vi "comm termination.vi"(8 "error in (no error)":errorcluster, 9 "termination characters":string, 10 "Termination Character Enable":bool, 11 "Comm Handle":u32) -> (0 "error out":errorcluster, 3 "dup Comm Handle":u32)   [LabVIEW 2017, in "lvserial.lvlib"]
doc: "Configures the termiation characters for the serial port."
uses:
  lvserial.lvlib
  lvserial.dll
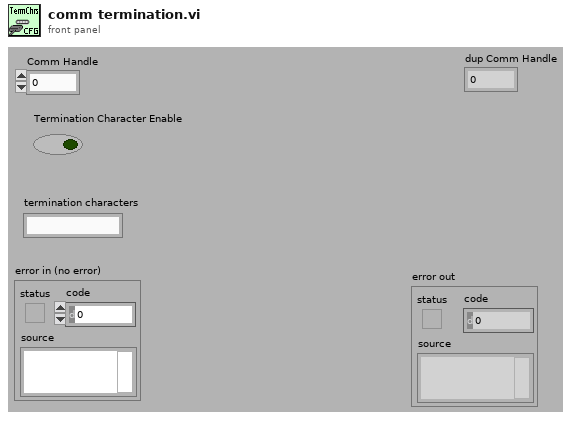
[diagram p1: front panel]
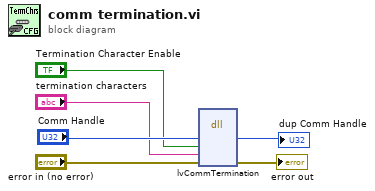
[diagram p0: block diagram]
diagram:
  n1 = dll-call lib="lvserial.dll" fn="lvCommTermination"("hComm"="Comm Handle", "Termination Character Enable"="Termination Character Enable", "pcTermCharacter"="termination characters", "error in (no error)"="error in (no error)") -> ("hComm"=→"dup Comm Handle":u32, "error in (no error)"=→"error out":errorcluster)  [unwired: 5 in, 3 out]
